vi "three ramps disorder.vi"(4 "P2 y":dbl, 5 "P1 y":dbl, 6 "P2 x":dbl, 7 "P1 x":dbl, 10 "level":dbl, 11 "points":i32) -> (3 "Array":dbl[](array[numeric]))   [LabVIEW 2023]
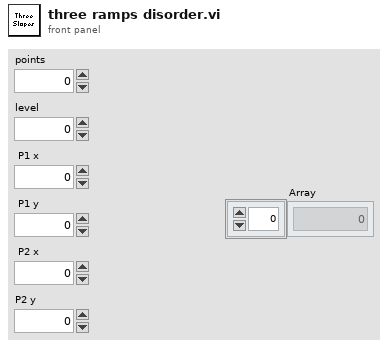
[diagram p1: front panel]
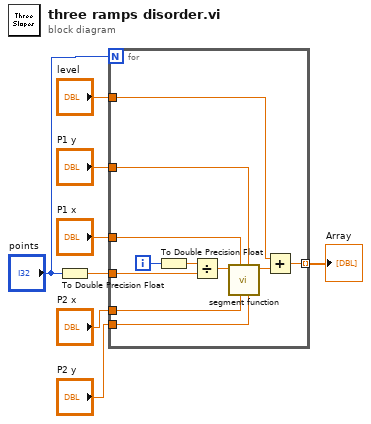
[diagram p0: block diagram]
diagram:
  n1 = To Double Precision Float(number="points") -> (double precision float=w7:dbl)
  n2 = for {
    N: "points" -> [_]
    tunnel: w7 -> [w17]
    tunnel: "P1 x" -> [w15]
    tunnel: "P1 y" -> [w14]
    tunnel: "P2 x" -> [w13]
    tunnel: "P2 y" -> [w12]
    tunnel: [w9] -> w2 mode=indexing
    tunnel: "level" -> [w10]
    i -> [w19]
    n3 = To Double Precision Float(number=w19) -> (double precision float=w18:dbl)
    n4 = Divide(x=w18, y=w17) -> (x/y=w16:dbl)
    n5 = call "segment function.vi"("y2"=w12, "y1"=w14, "x2"=w13, "x1"=w15, "x"=w16) -> ("y"=w11:dbl)  [unwired: 6 in]
    n6 = Add(x=w10, y=w11) -> (x+y=w9:dbl)
  }
  "Array" <- w2
